vi "VMI_image_display.vi"(0 "Image_control":refnum<vi>, 1 "Image to show":u16, 2 "Current Image":i32[][](array[numeric]), 4 "Big_image Array":i16[][][](array[numeric]), 5 "Canvas":T1) -> (7 "Image_out":T1(plugin-control))   [LabVIEW 2018]
uses:
  <vilib>/vision/Image Controls.llb/IMAQ Image.ctl
panel:
  in  "Real Time":T1(plugin-control)=refnum
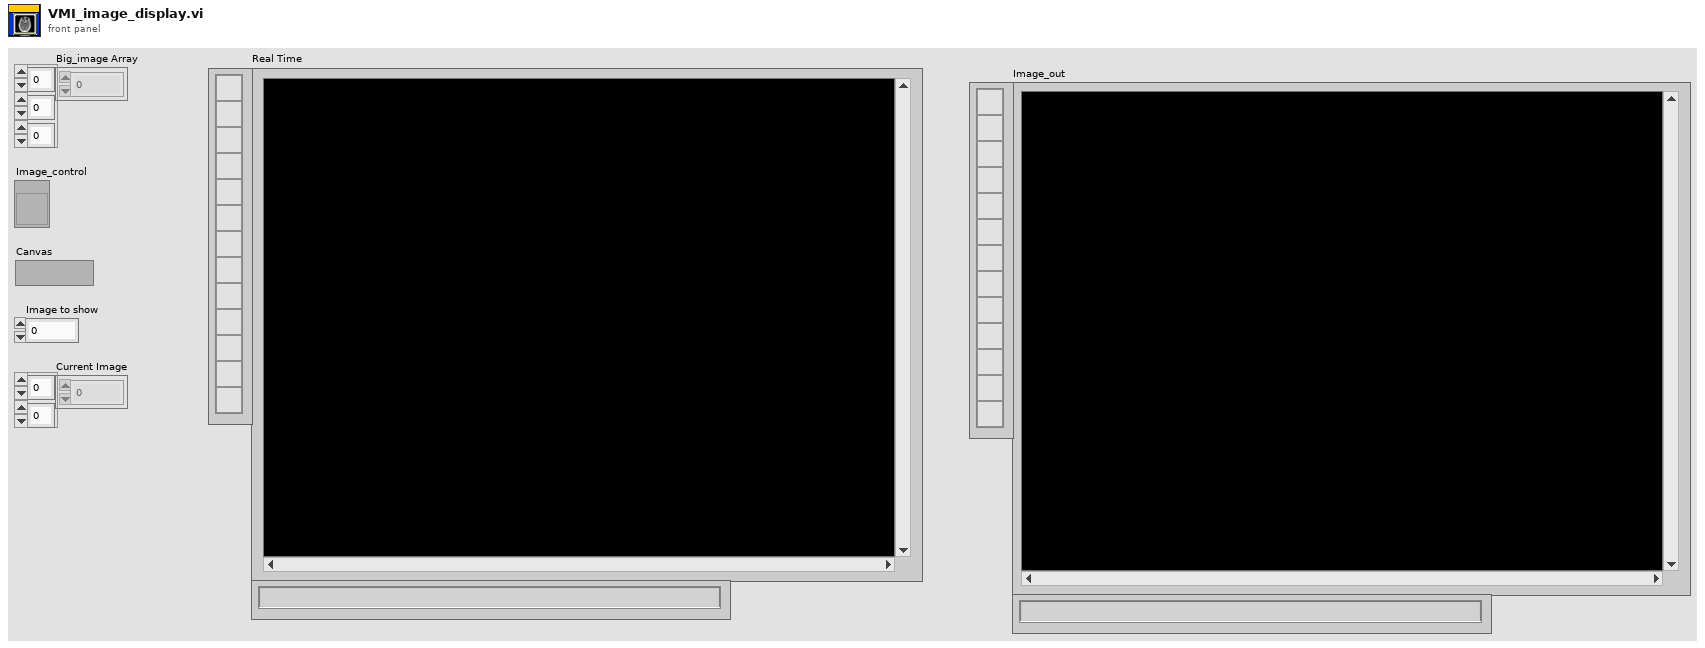
[diagram p1: front panel]
types:
  T1 = typedef "IMAQ Image.ctl" = refnum<image>
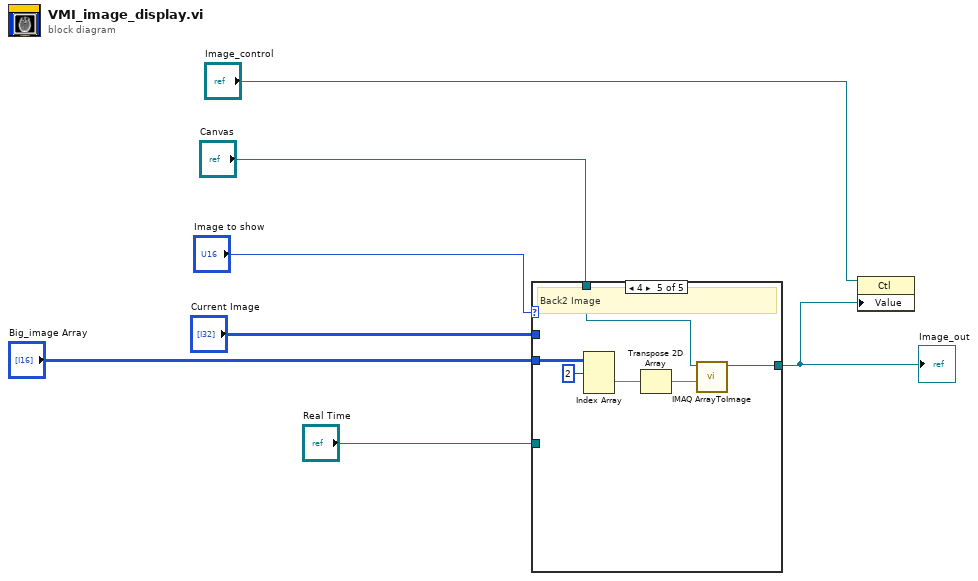
[diagram p0: block diagram]
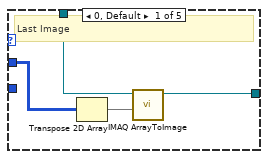
[diagram p2: hidden frame]
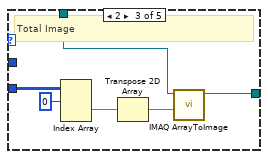
[diagram p4: hidden frame]
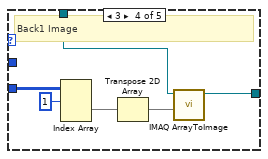
[diagram p5: hidden frame]
diagram:
  n1 = case shown="4" "Image to show" {
    tunnel: "Current Image" -> [w10 _ _ _ _]
    tunnel: "Canvas" -> [w9 _ w13 w19 w25]
    tunnel: "Big_image Array" -> [_ _ w16 w22 w28]
    tunnel: [w8 w12 w17 w23 w29] -> w3
    tunnel: "Real Time" -> [_ w12 _ _ _]
    frame 0, Default {
      # "Last Image"
      n2 = Transpose 2D Array(2D array=w10) -> (transposed array=w11:i32[][])
      n3 = call "IMAQ ArrayToImage"("Image Pixels (I16)"=w11, "Image"=w9) -> ("Image Out"=w8:T1)  [unwired: 8 in, 1 out]
    }
    frame 1 {
      # "Real Time"
    }
    frame 2 {
      # "Total Image"
      n4 = Index Array(array=w16, index (dim 0)=0 ("index (page)")) -> (element=w15:i16[][])  [unwired: 2 in]
      n5 = Transpose 2D Array(2D array=w15) -> (transposed array=w18:i16[][])
      n6 = call "IMAQ ArrayToImage"("Image Pixels (I16)"=w18, "Image"=w13) -> ("Image Out"=w17:T1)  [unwired: 8 in, 1 out]
    }
    frame 3 {
      # "Back1 Image"
      n7 = Index Array(array=w22, index (dim 0)=1 ("index (page)")) -> (element=w21:i16[][])  [unwired: 2 in]
      n8 = Transpose 2D Array(2D array=w21) -> (transposed array=w24:i16[][])
      n9 = call "IMAQ ArrayToImage"("Image Pixels (I16)"=w24, "Image"=w19) -> ("Image Out"=w23:T1)  [unwired: 8 in, 1 out]
    }
    frame 4 {
      # "Back2 Image"
      n10 = Index Array(array=w28, index (dim 0)=2 ("index (page)")) -> (element=w27:i16[][])  [unwired: 2 in]
      n11 = Transpose 2D Array(2D array=w27) -> (transposed array=w30:i16[][])
      n12 = call "IMAQ ArrayToImage"("Image Pixels (I16)"=w30, "Image"=w25) -> ("Image Out"=w29:T1)  [unwired: 8 in, 1 out]
    }
  }
  "Image_out" <- w3
  n13 = property class="Ctl"(reference="Image_control", "Value"=w3) -> ()  [unwired: 1 in, 2 out]
